vi "Cross-Talk, Process Pulses.vi"(8 "error in":errorcluster, 10 "Resistance Array (ohms)":dbl[](array[numeric]), 11 "Waveform Array":waveform(dbl)[](array[waveform])) -> (0 "error out":errorcluster, 3 "Amplitudes Out (uA)":dbl[](array[numeric]))   [LabVIEW 2010]
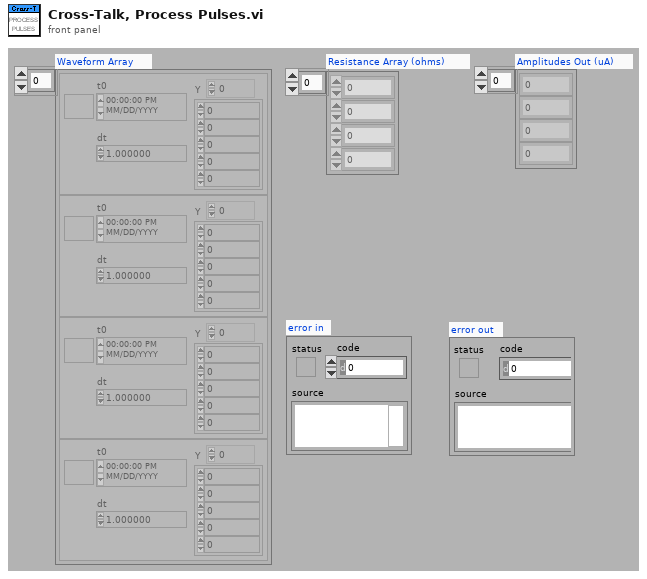
[diagram p1: front panel]
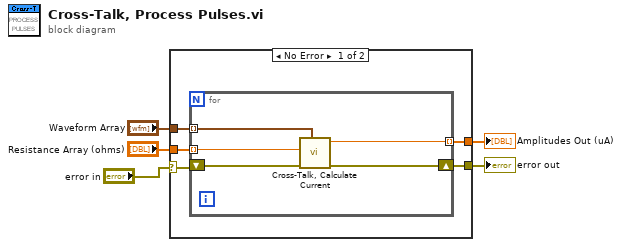
[diagram p0: block diagram]
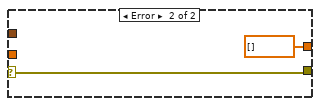
[diagram p2: hidden frame]
diagram:
  n1 = case shown="No Error" "error in" {
    selector: "error in" -> [w6 w17]
    tunnel: "Waveform Array" -> [w10 _]
    tunnel: "Resistance Array (ohms)" -> [w9 _]
    tunnel: [w8 dbl[] []] -> w3
    tunnel: [w7 w17] -> w2
    frame No Error {
      n2 = for {
        tunnel: w10 -> [w14] mode=indexing
        tunnel: w9 -> [w15] mode=indexing
        tunnel: [w13] -> w8 mode=indexing
        shift-right: [w12] -> w7
        shift-left: w6 -> [w11]
        n3 = call "Cross-Talk, Calculate Current.vi"("Waveform In"=w14, "error in"=w11, "Resistance (ohms)"=w15) -> ("error out"=w12:errorcluster, "Amplitude (uA)"=w13:dbl)  [unwired: 7 in]
      }
    }
    frame Error {
    }
  }
  "Amplitudes Out (uA)" <- w3
  "error out" <- w2
